vi "VIPM package installation automation.vi"() -> ()   [LabVIEW 2016]
uses:
  <vilib>/JKI/VIPM API/VIPM API_vipm_api.lvlib
panel:
  out "error out":errorcluster
  in  "Error In":errorcluster
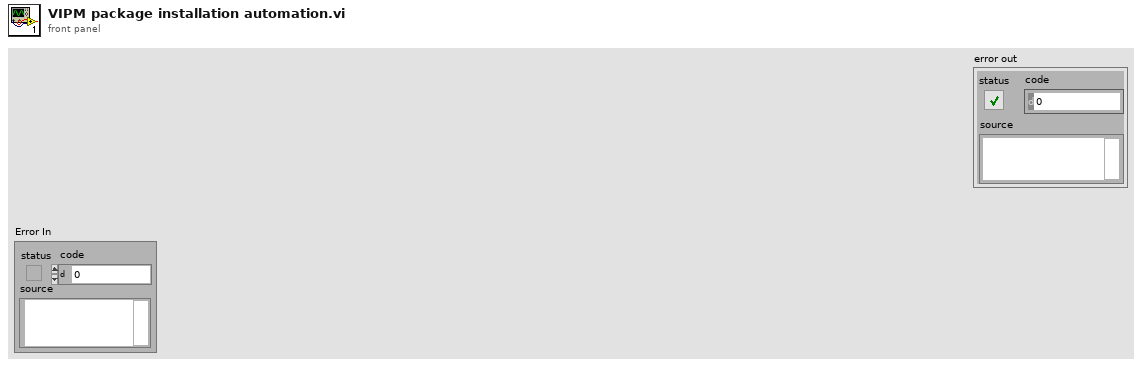
[diagram p1: front panel]
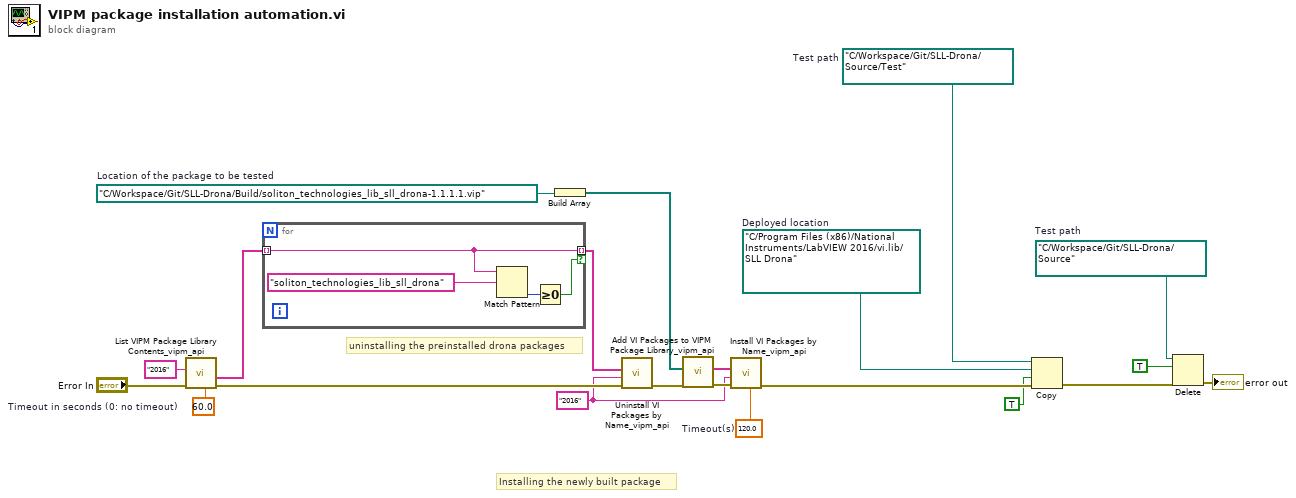
[diagram p0: block diagram]
diagram:
  w4 = path "C:/Workspace/Git/SLL-Drona/Source/Test"  # Test path
  w6 = 120.0  # Timeout(s)
  w11 = path "C:/Workspace/Git/SLL-Drona/Build/soliton_technologies_lib_sll_drona-1.1.1.1.vip"  # Location of the package to be tested
  w15 = 60.0  # Timeout in seconds (0: no timeout)
  w7 = "2016" ("LabVIEW Version")
  w18 = path "C:/Workspace/Git/SLL-Drona/Source"  # Test path
  w21 = path "C:/Program Files (x86)/National Instruments/LabVIEW 2016/vi.lib/SLL Drona"  # Deployed location
  # "uninstalling the preinstalled drona packages"
  # "Installing the newly built package"
  n1 = call <vilib>:"List VIPM Package Library Contents_vipm_api.vi"("Timeout in seconds (0: no timeout)"=w15, "error in (no error)"="Error In", "LabVIEW Version"="2016") -> ("error out"=w13:errorcluster, "Package Names []"=w14:string[])  [unwired: 6 in, 1 out]
  n2 = for {
    tunnel: w14 -> [w23] mode=indexing
    tunnel: [w23] -> w12 mode=indexing if=w22
    n3 = Match Pattern(string=w23, regular expression="soliton_technologies_lib_sll_drona") -> (offset past match=w24:i32)  [unwired: 1 in, 3 out]
    n4 = Greater Or Equal To 0?(x=w24) -> (x >= 0?=w22:bool)
  }
  n5 = Build Array(w11) -> (w10:path[])
  n6 = call <vilib>:"Uninstall VI Packages by Name_vipm_api.vi"("error in (no error)"=w13, "LabVIEW Version"=w7, "Package Names to Uninstall []"=w12) -> ("error out"=w17:errorcluster)  [unwired: 8 in]
  n7 = call <vilib>:"Add VI Packages to VIPM Package Library_vipm_api.vi"("error in (no error)"=w17, "Packages to add to VIPM Library (vipc,vip,ogp)"=w10) -> ("error out"=w9:errorcluster, "Package Names Added"=w8:string[])  [unwired: 8 in]
  n8 = call <vilib>:"Install VI Packages by Name_vipm_api.vi"("Timeout in seconds (0: no timeout)"=w6, "error in (no error)"=w9, "LabVIEW Version"=w7, "Package Names to Install []"=w8) -> ("error out"=w20:errorcluster)  [unwired: 7 in]
  n9 = Copy(8:w20, 9:TRUE ("overwrite (F)"), 10:w21, 11:w4) -> (0:w19:errorcluster)  [unwired: 1 in, 2 out]
  n10 = Delete(path (use dialog)=w18, entire hierarchy (F)=TRUE, error in=w19) -> (error out=→"error out":errorcluster)  [unwired: 2 in, 2 out]
